vi "Periodic Tasks.vi"   [LabVIEW 2012]
doc: "This VI runs in parallel to other tasks. It can contain as many user-defined periodic loops as you need. These can carry out PID or other sorts of timed response."
uses:
  <vilib>/Rock Robotics/SystemInterfaces/Utilities/FPGA_UtilitiesLED Source.ctl
  <vilib>/Rock Robotics/SystemInterfaces/Utilities/FPGA_UtilitiesLED State.ctl
  Robot Global Data.vi
types:
  T1 = typedef "FPGA_UtilitiesLED State.ctl" = enum16{"Off", "On", "Toggle"}
  T2 = typedef "FPGA_UtilitiesLED Source.ctl" = enum16{"User LED", "FPGA LED"}
  T3 = cluster{"Case":dbl, "VisionTrack":bool, "ShootEnableWheels":bool, "Shoot":bool, "ManualExtend":dbl, "ManualRotate":dbl, "YCoord":dbl, "FlipUp":bool, "RotDeadband":dbl, "ExtDeadband":dbl, "ExtPOT":dbl, "RotPOT":dbl, "WheelFSpd":dbl, "WheelBSpd":dbl, "ServoPositions":cluster{"FlipperLeftUp":dbl, "FlipperLeftDown":dbl, "FlipperRightUp":dbl, "FlipperRightDown":dbl, "KickerLeftBack":dbl, "KickerLeftForward":dbl, "KickerRightBack":dbl, "KickerRightForward":dbl}, "POTPositions":cluster{"Setpoint 1":dbl, "Setpoint 2":dbl, "Setpoint 3":dbl, "Setpoint 4":dbl, "RotLow":dbl, "RotHigh":dbl, "ExtLow":dbl, "ExtHigh":dbl}, "ClimberHooked":bool}
  T4 = cluster{"FlipperLeftUp":dbl, "FlipperLeftDown":dbl, "FlipperRightUp":dbl, "FlipperRightDown":dbl, "KickerLeftBack":dbl, "KickerLeftForward":dbl, "KickerRightBack":dbl, "KickerRightForward":dbl}
  T5 = cluster{"Setpoint 1":dbl, "Setpoint 2":dbl, "Setpoint 3":dbl, "Setpoint 4":dbl, "RotLow":dbl, "RotHigh":dbl, "ExtLow":dbl, "ExtHigh":dbl}
  T6 = typedef "WPI_AnalogChannelDevRef.ctl" = cluster{"DevStatus":errorcluster, "Analog Module":T7, "Analog Channel":T8}
  T7 = typedef "FPGA_TypedefAnalogModule.ctl" = enum16{"Analog Module 1", "Analog Module 2"}
  T8 = typedef "FPGA_AIChannel.ctl" = enum8{"AI 1", "AI 2", "AI 3", "AI 4", "AI 5", "AI 6", "AI 7", "AI 8", "Invalid"}
  T9 = typedef "WPI_DigitalInputDevRef.ctl" = cluster{"DevStatus":errorcluster, "DIO Channel":T10, "Digital Module":T11}
  T10 = typedef "FPGA_DIOChannel.ctl" = enum8{"DIO 1", "DIO 2", "DIO 3", "DIO 4", "DIO 5", "DIO 6", "DIO 7", "DIO 8", "DIO 9", "DIO 10", "DIO 11", "DIO 12", "DIO 13", "DIO 14", "Invalid"}
  T11 = typedef "FPGA_TypedefDigitalModule.ctl" = enum16{"Digital Module 1", "Digital Module 2"}
  T12 = typedef "WPI_RelayValue.ctl" = enum16{"Off", "On", "Forward", "Reverse"}
  T13 = cluster{"Case":dbl, "Extension":dbl, "Rotation":dbl, "WheelF":dbl, "WheelB":dbl, "Left Kicker":dbl, "Right Kicker":dbl, "Left Flipper":dbl, "Right Flipper":dbl, "Lights":T12}
  T14 = typedef "WPI_GyroDevRef.ctl" = cluster{"DevStatus":errorcluster, "Analog Module":T7, "Analog Channel":T8, "Offset":dbl, "Gain (VoltsPerDegree/Second)":dbl}
  T15 = typedef "WPI_EncoderDevRef.ctl" = cluster{"DevStatus":errorcluster, "EncoderIndex":T16, "CounterIndex":T17, "DistancePerCount":dbl, "Decoding Type":T18}
  T16 = typedef "FPGA_EncoderIdx.ctl" = enum8{"Enc 0", "Enc 1", "Enc 2", "Enc 3", "Invalid"}
  T17 = typedef "FPGA_CounterCtrSystemIndex.ctl" = enum8{"Ctr 0", "Ctr 1", "Ctr 2", "Ctr 3", "Ctr 4", "Ctr 5", "Ctr 6", "Ctr 7", "Invalid"}
  T18 = typedef "WPI_EncoderType.ctl" = enum16{"1x", "2x", "4x"}
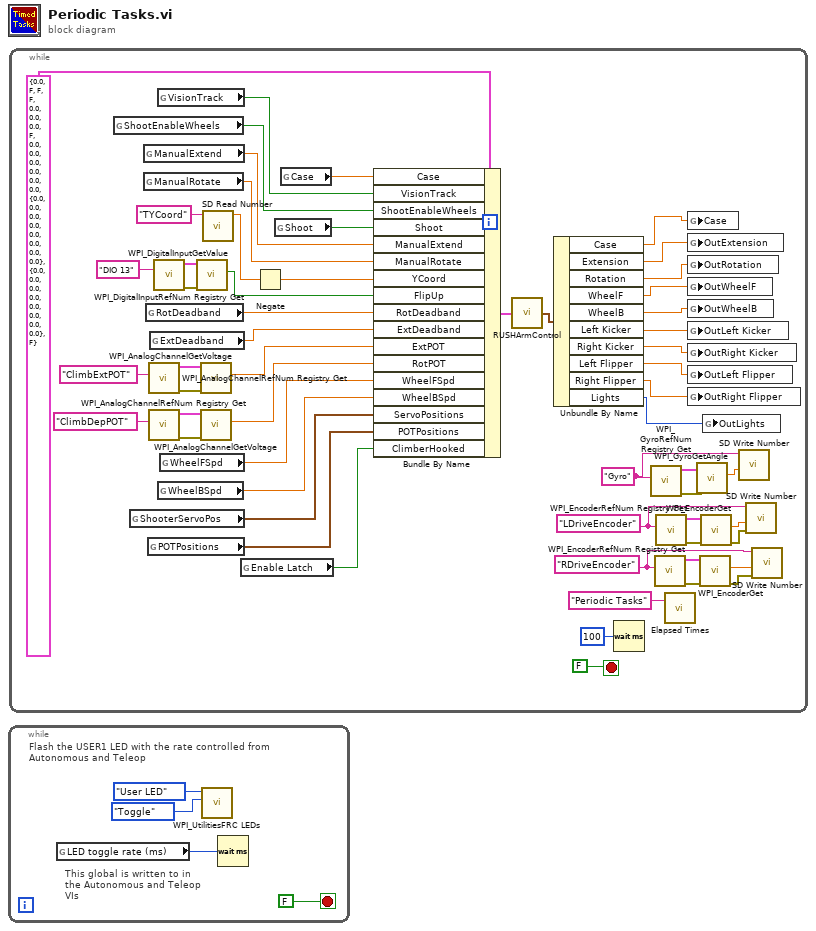
[diagram p0: block diagram]
diagram:
  n1 = while {
    stop <- FALSE stop-if-true
    # "This global is written to in the Autonomous and Teleop VIs"
    # "Flash the USER1 LED with the rate controlled from Autonomous and Teleop"
    n2 = global read "Robot Global Data.vi" "LED toggle rate (ms)"() -> (w1:u32)
    n3 = call <vilib>:"WPI_UtilitiesFRC LEDs.vi"("State"=FPGA_UtilitiesLED_State."Toggle", "LED Type"=FPGA_UtilitiesLED_Source."User LED") -> ()  [unwired: 1 in, 9 out]
    n4 = Wait (ms)(milliseconds to wait=w1) -> ()  [unwired: 1 out]
  }
  n5 = while {
    stop <- FALSE stop-if-true
    w19 = "RDriveEncoder" ("refnum name")
    w15 = "LDriveEncoder" ("refnum name")
    w13 = "Gyro" ("refnum name")
    n6 = global read "Robot Global Data.vi" "ShootEnableWheels"() -> (w43:bool)
    n7 = global read "Robot Global Data.vi" "ShooterServoPos"() -> (w35:T4)
    n8 = global read "Robot Global Data.vi" "ManualExtend"() -> (w41:dbl)
    n9 = global read "Robot Global Data.vi" "ManualRotate"() -> (w40:dbl)
    n10 = global read "Robot Global Data.vi" "RotDeadband"() -> (w39:dbl)
    n11 = global read "Robot Global Data.vi" "POTPositions"() -> (w34:T5)
    n12 = call <vilib>:"WPI_AnalogChannelRefNum Registry Get.vi"("refnum name"="ClimbExtPOT") -> ("error out"=w57:errorcluster, "AIDeviceRef"=w56:T6)  [unwired: 9 in]
    n13 = call <vilib>:"WPI_AnalogChannelRefNum Registry Get.vi"("refnum name"="ClimbDepPOT") -> ("error out"=w51:errorcluster, "AIDeviceRef"=w50:T6)  [unwired: 9 in]
    n14 = global read "Robot Global Data.vi" "ExtDeadband"() -> (w38:dbl)
    n15 = call <vilib>:"WPI_DigitalInputRefNum Registry Get.vi"("refnum name"="DIO 13") -> ("error out"=w10:errorcluster, "DigitalInputDevRef"=w9:T9)  [unwired: 9 in]
    n16 = global read "Robot Global Data.vi" "VisionTrack"() -> (w44:bool)
    n17 = global read "Robot Global Data.vi" "WheelBSpd"() -> (w36:dbl)
    n18 = global read "Robot Global Data.vi" "WheelFSpd"() -> (w37:dbl)
    n19 = call <vilib>:"WPI_DigitalInputGetValue.vi"("error in (no error)"=w10, "DigitalInputDevRef"=w9) -> ("Value"=w7:bool)  [unwired: 7 in, 2 out]
    n20 = call <vilib>:"WPI_AnalogChannelGetVoltage.vi"("error in (no error)"=w57, "AIDeviceRef"=w56) -> ("Voltage"=w31:dbl)  [unwired: 7 in, 2 out]
    n21 = call <vilib>:"WPI_AnalogChannelGetVoltage.vi"("error in (no error)"=w51, "AIDeviceRef"=w50) -> ("Voltage"=w30:dbl)  [unwired: 7 in, 2 out]
    n22 = call <vilib>:"SD Read Number.vi"("Name"="TYCoord") -> ("Numeric"=w6:dbl)  [unwired: 8 in, 2 out]
    n23 = global read "Robot Global Data.vi" "Enable Latch"() -> (w11:bool)
    n24 = Negate(x=w6) -> (-x=w5:dbl)
    n25 = global read "Robot Global Data.vi" "Shoot"() -> (w42:bool)
    n26 = global read "Robot Global Data.vi" "Case"() -> (w45:dbl)
    n27 = Bundle By Name(cluster=T3 {"Case"=0.0, "VisionTrack"=FALSE, "ShootEnableWheels"=FALSE, "Shoot"=FALSE, "ManualExtend"=0.0, "ManualRotate"=0.0, "YCoord"=0.0, "FlipUp"=FALSE, "RotDeadband"=0.0, "ExtDeadband"=0.0, "ExtPOT"=0.0, "RotPOT"=0.0, "WheelFSpd"=0.0, "WheelBSpd"=0.0, "ServoPositions"={"FlipperLeftUp"=0.0, "FlipperLeftDown"=0.0, "FlipperRightUp"=0.0, "FlipperRightDown"=0.0, "KickerLeftBack"=0.0, "KickerLeftForward"=0.0, "KickerRightBack"=0.0, "KickerRightForward"=0.0}, "POTPositions"={"Setpoint 1"=0.0, "Setpoint 2"=0.0, "Setpoint 3"=0.0, "Setpoint 4"=0.0, "RotLow"=0.0, "RotHigh"=0.0, "ExtLow"=0.0, "ExtHigh"=0.0}, "ClimberHooked"=FALSE} ("In Cluster"), "Case"=w45, "VisionTrack"=w44, "ShootEnableWheels"=w43, "Shoot"=w42, "ManualExtend"=w41, "ManualRotate"=w40, "YCoord"=w5, "FlipUp"=w7, "RotDeadband"=w39, "ExtDeadband"=w38, "ExtPOT"=w31, "RotPOT"=w30, "WheelFSpd"=w37, "WheelBSpd"=w36, "ServoPositions"=w35, "POTPositions"=w34, "ClimberHooked"=w11) -> (w47:T3)
    n28 = call "RUSHArmControl.vi"("In Cluster"=w47) -> ("Out Cluster"=w46:T13)
    n29 = Unbundle By Name(w46) -> ("Case"=w29:dbl, "Extension"=w28:dbl, "Rotation"=w27:dbl, "WheelF"=w26:dbl, "WheelB"=w25:dbl, "Left Kicker"=w24:dbl, "Right Kicker"=w23:dbl, "Left Flipper"=w22:dbl, "Right Flipper"=w21:dbl, "Lights"=w12:T12)
    n30 = Wait (ms)(milliseconds to wait=u32 100) -> ()  [unwired: 1 out]
    n31 = call <vilib>:"WPI_GyroRefNum Registry Get.vi"("refnum name"=w13) -> ("error out"=w58:errorcluster, "GyroDevRef"=w59:T14)  [unwired: 9 in]
    n32 = call <vilib>:"WPI_EncoderRefNum Registry Get.vi"("refnum name"=w19) -> ("error out"=w53:errorcluster, "EncoderDevRef"=w52:T15)  [unwired: 9 in]
    n33 = call <vilib>:"WPI_EncoderRefNum Registry Get.vi"("refnum name"=w15) -> ("error out"=w54:errorcluster, "EncoderDevRef"=w55:T15)  [unwired: 9 in]
    n34 = call "Elapsed Times.vi"("Call Name"="Periodic Tasks") -> ()  [unwired: 2 in, 1 out]
    n35 = global write "Robot Global Data.vi" "Case"(w29) -> ()
    n36 = global write "Robot Global Data.vi" "OutExtension"(w28) -> ()
    n37 = global write "Robot Global Data.vi" "OutRotation"(w27) -> ()
    n38 = global write "Robot Global Data.vi" "OutWheelF"(w26) -> ()
    n39 = global write "Robot Global Data.vi" "OutWheelB"(w25) -> ()
    n40 = global write "Robot Global Data.vi" "OutLeft Kicker"(w24) -> ()
    n41 = global write "Robot Global Data.vi" "OutRight Kicker"(w23) -> ()
    n42 = global write "Robot Global Data.vi" "OutLeft Flipper"(w22) -> ()
    n43 = global write "Robot Global Data.vi" "OutRight Flipper"(w21) -> ()
    n44 = call <vilib>:"WPI_GyroGetAngle.vi"("error in (no error)"=w58, "GyroDevRef"=w59) -> ("Angle"=w14:dbl)  [unwired: 6 in, 3 out]
    n45 = call <vilib>:"WPI_EncoderGet.vi"("error in (no error)"=w53, "EncoderDevRef"=w52) -> ("error out"=w16:errorcluster, "Distance"=w20:dbl)  [unwired: 4 in, 4 out]
    n46 = call <vilib>:"WPI_EncoderGet.vi"("error in (no error)"=w54, "EncoderDevRef"=w55) -> ("error out"=w18:errorcluster, "Distance"=w17:dbl)  [unwired: 4 in, 4 out]
    n47 = global write "Robot Global Data.vi" "OutLights"(w12) -> ()
    n48 = call <vilib>:"SD Write Number.vi"("Numeric"=w14, "Name"=w13) -> ()  [unwired: 8 in, 2 out]
    n49 = call <vilib>:"SD Write Number.vi"("error in"=w18, "Numeric"=w17, "Name"=w15) -> ()  [unwired: 7 in, 2 out]
    n50 = call <vilib>:"SD Write Number.vi"("error in"=w16, "Numeric"=w20, "Name"=w19) -> ()  [unwired: 7 in, 2 out]
  }
